vi "test_TrajectoryMH100122AODRAPS.vi"() -> ()   [LabVIEW 2010, in "TrajectoryMH100122AODRAPS.lvclass"]
uses:
  TrajectoryMH100122AODRAPS.lvclass
  raps_points_cluster.ctl
  common/classes/ErrorController/ErrorController/ErrorController.lvclass
  TrajectoryMH100122AODRAPS.lvclass/TrajectoryMH100122AODRAPS.ctl
  common/classes/ErrorController/ErrorController/class_data.vi
panel:
  in  "RAPS points cluster":T1
  out "error loaded?":bool
  in  "Define":bool
  in  "initialise":bool
  in  "number of frames":i32
  in  "startButton":bool
  in  "createButton":bool
  in  "repetition rate":dbl[unit]=10.0
  in  "stop":bool
  # "Test VI for TrajectoryMH100122AODRAPS"
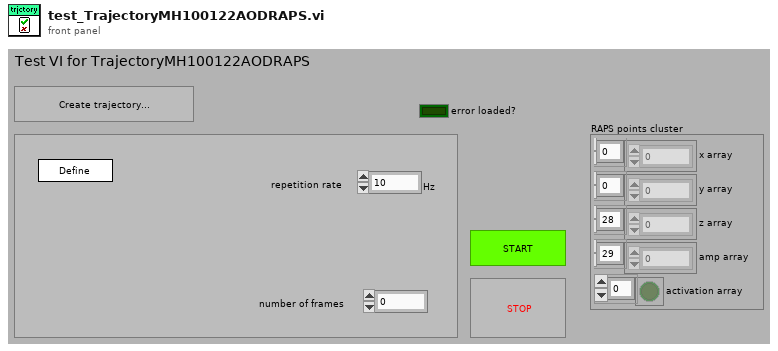
[diagram p1: front panel]
types:
  T1 = typedef "TrajectoryMH100122AODRAPS.lvclass/raps_points_cluster.ctl" = cluster{"x array":u16[], "y array":u16[], "z array":u16[], "amp array":u16[], "activation array":bool[]}
  T2 = typedef "plugin_specification.ctl" = cluster{"class path":string, "configuration":string, "label":string, "settings name":string}
  T3 = typedef "XComponentSpecification.xctl/data.ctl" = cluster{"class path":string, "configuration":string, "label":string, "settings name":string}
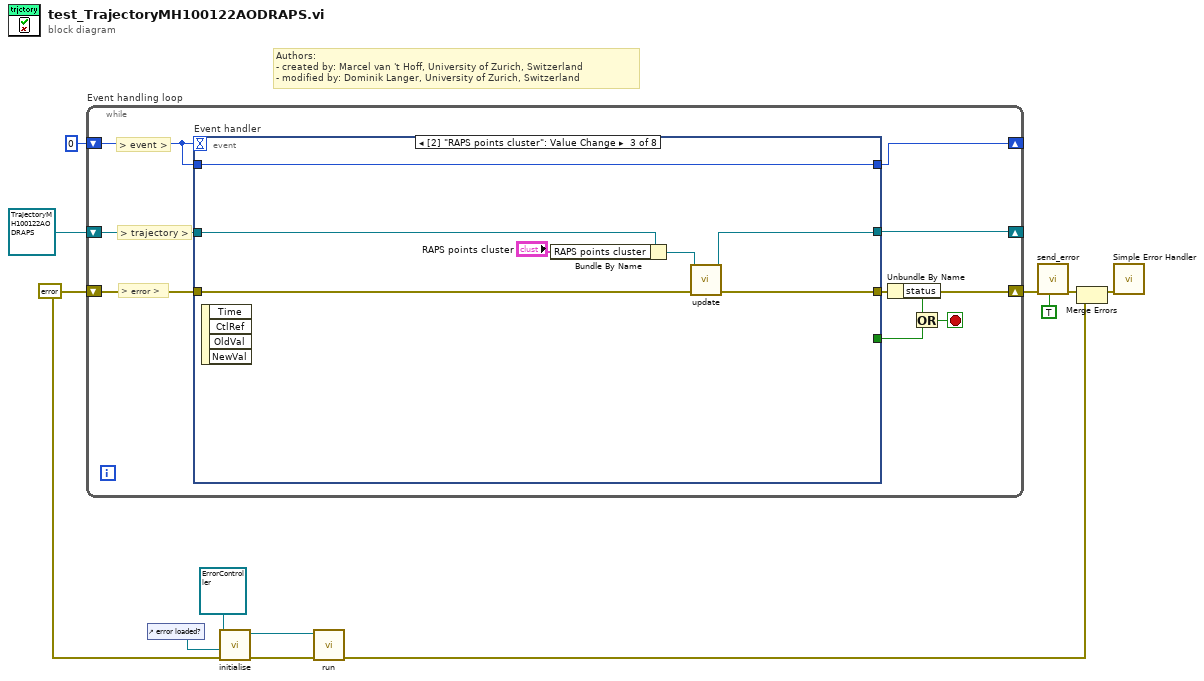
[diagram p0: block diagram]
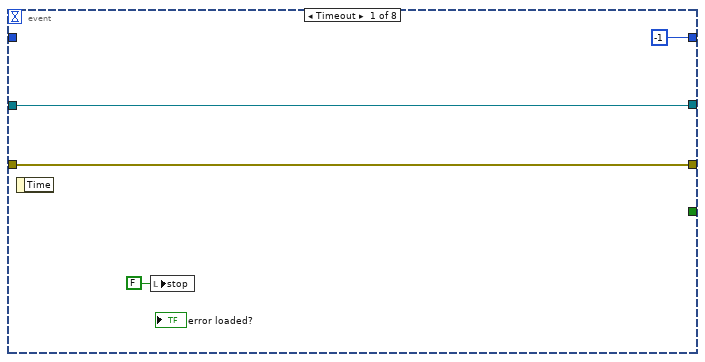
[diagram p2: hidden frame]
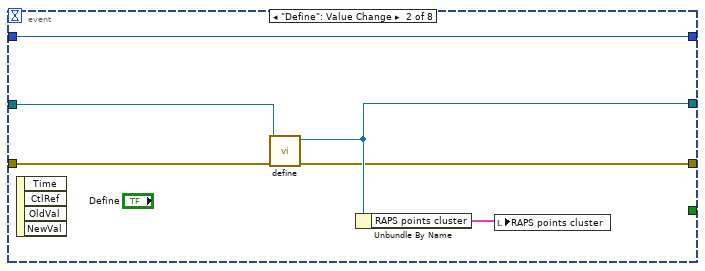
[diagram p3: hidden frame]
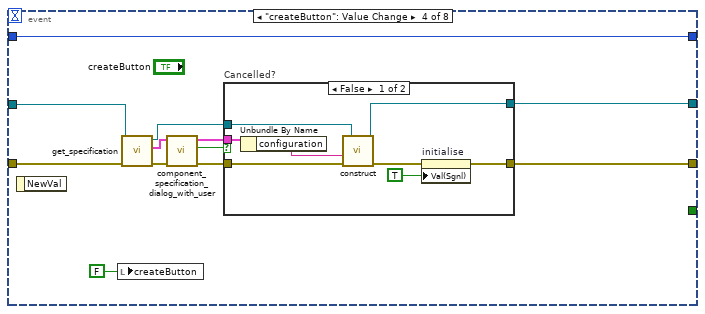
[diagram p4: hidden frame]
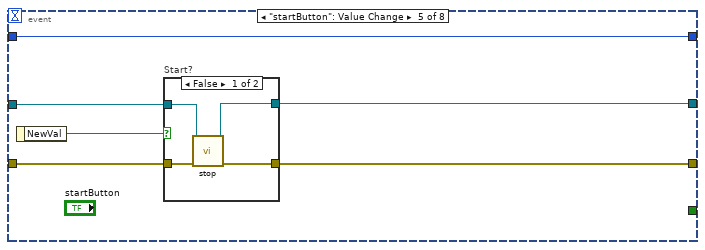
[diagram p6: hidden frame]
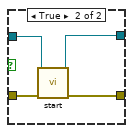
[diagram p7: hidden frame]
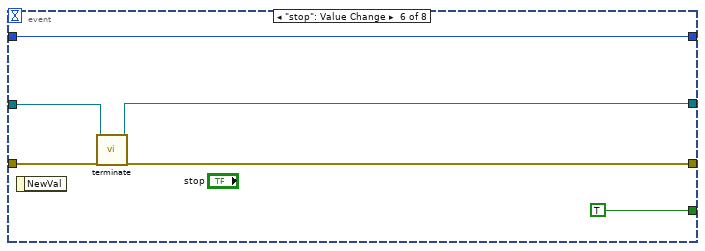
[diagram p8: hidden frame]
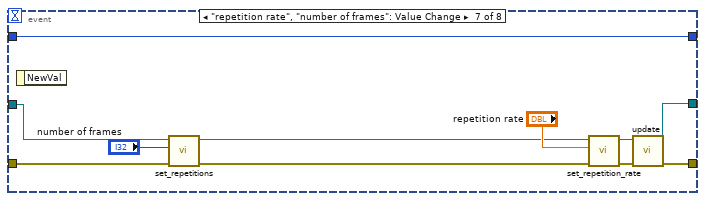
[diagram p9: hidden frame]
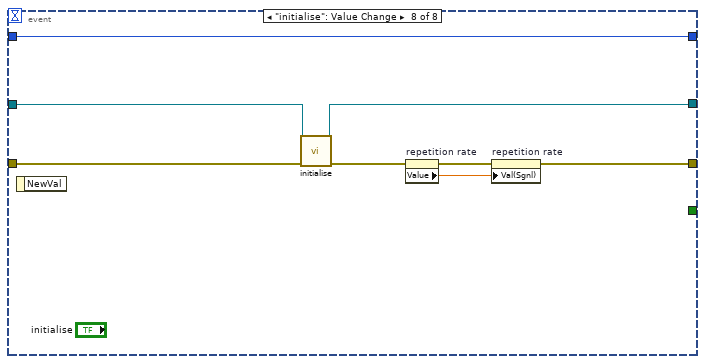
[diagram p10: hidden frame]
diagram:
  w8 = errorcluster {"status"=FALSE, "code"=0, "source"=""} ("error out")
  # "Authors: \n- created by: Marcel van 't Hoff, University of Zurich, Switzerland\n- modified by: Dominik Langer, University of Zurich, Switzerland"
  n1 = while "Event handling loop" {
    shift-right: [w14] -> _
    shift-left: 0 -> [w13]
    shift-right: [w18] -> w3
    shift-left: w8 -> [w21]
    shift-right: [w19] -> _
    shift-left: refnum<class "TrajectoryMH100122AODRAPS.lvclass"> refnum ("TrajectoryMG100122AODFrameScan.lvclass") -> [w20]
    stop <- w16 stop-if-true
    # "> trajectory >"
    # "> error >"
    # "> event >"
    n2 = event "Event handler" shown="[2] \"RAPS points cluster\": Value Change" {
      selector: _ -> [_ _ _ _ _ _ _ _]
      dyn-events: _ -> [_ _ _ _ _ _ _ _]
      timeout: w13 -> [_ _ _ _ _ _ _ _]
      tunnel: [-1 w31 w38 w50 w66 w79 w91 w99] -> w14
      tunnel: w13 -> [_ w31 w38 w50 w66 w79 w91 w99]
      tunnel: [w23 w26 w36 w47 w63 w77 w87 w92] -> w18
      tunnel: w21 -> [w23 w29 w37 w44 w64 w78 w89 w98]
      tunnel: [w24 w27 w35 w48 w62 w75 w86 w96] -> w19
      tunnel: w20 -> [w24 w30 w34 w42 w65 w76 w88 w97]
      tunnel: [_ _ _ _ _ TRUE ("stop") _ _] -> w15
      event Timeout {
        n3 = event-data() -> ()  [unwired: 1 in, 1 out]
        n4 = local write "stop"(FALSE ("stop")) -> ()
      }
      event "Define": Value Change {
        n5 = event-data() -> ()  [unwired: 1 in, 4 out]
        n6 = call-dynamic "define.vi"("error in (no error)"=w29, "TrajectoryMH100122AODRAPS in"=w30) -> ("error out"=w26:errorcluster, "TrajectoryMH100122AODRAPS out"=w27:refnum<class "TrajectoryMH100122AODRAPS.lvclass">)  [unwired: 8 in]
        n7 = Unbundle By Name(w27) -> ("RAPS points cluster"=w28:T1)
        n8 = local write "RAPS points cluster"(w28) -> ()
      }
      event Value Change {
        n9 = event-data() -> ()  [unwired: 1 in, 4 out]
        n10 = Bundle By Name(cluster=w34, "RAPS points cluster"="RAPS points cluster") -> (w33:refnum<class "TrajectoryMH100122AODRAPS.lvclass">)
        n11 = call-dynamic "update.vi"("error in (no error)"=w37, "TrajectoryMG100122AODFrameScan in"=w33) -> ("error out"=w36:errorcluster, "TrajectoryMG100122AODFrameScan out"=w35:refnum<class "TrajectoryMH100122AODRAPS.lvclass">)  [unwired: 8 in]
      }
      event "createButton": Value Change {
        n12 = event-data() -> ()  [unwired: 1 in, 1 out]
        n13 = local write "createButton"(FALSE ("createButton")) -> ()
        n14 = call-dynamic "get_specification.vi"("error in (no error)"=w44, "GenericPlugin in"=w42) -> ("error out"=w45:errorcluster, "component specification"=w46:T2, "GenericPlugin out"=w41:refnum<class "TrajectoryMH100122AODRAPS.lvclass">)  [unwired: 6 in, 1 out]
        n15 = call "component_specification_dialog_with_user.vi"("error in (no error)"=w45, "component specification in"=w46) -> ("error out"=w43:errorcluster, "cancelled?"=w39:bool, "component specification out"=w40:T3)  [unwired: 7 in]
        n16 = case "Cancelled?" shown="False" w39 {
          tunnel: [w58 w59] -> w48
          tunnel: [w55 w60] -> w47
          tunnel: w43 -> [w54 w60]
          tunnel: w41 -> [w53 w59]
          tunnel: w40 -> [w52 _]
          frame False {
            n17 = Unbundle By Name(w52) -> ("configuration"=w51:string)
            n18 = call-dynamic "construct.vi"("error in (no error)"=w54, "configuration name"=w51, "GenericPlugin in"=w53) -> ("error out"=w56:errorcluster, "GenericPlugin out"=w58:refnum<class "TrajectoryMH100122AODRAPS.lvclass">)  [unwired: 7 in]
            n19 = property on="initialise" class="Bool (strict)"(error in=w56, "Val(Sgnl)"=TRUE ("Value (Signaling)")) -> (error out=w55:errorcluster)  [unwired: 1 in, 1 out]
          }
          frame True {
          }
        }
      }
      event "startButton": Value Change {
        n20 = event-data() -> ("NewVal"=w61:bool)  [unwired: 1 in]
        n21 = case "Start?" shown="False" w61 {
          tunnel: w65 -> [w68 w74]
          tunnel: w64 -> [w70 w73]
          tunnel: [w69 w72] -> w63
          tunnel: [w67 w71] -> w62
          frame False {
            n22 = call-dynamic "stop.vi"("error in (no error)"=w70, "TrajectoryMG100122GenericFPGA in"=w68) -> ("error out"=w69:errorcluster, "TrajectoryMG100122GenericFPGA out"=w67:refnum<class "TrajectoryMH100122AODRAPS.lvclass">)  [unwired: 8 in]
          }
          frame True {
            n23 = call-dynamic "start.vi"("error in (no error)"=w73, "TrajectoryMG100122GenericFPGA in"=w74) -> ("error out"=w72:errorcluster, "TrajectoryMG100122GenericFPGA out"=w71:refnum<class "TrajectoryMH100122AODRAPS.lvclass">)  [unwired: 8 in]
          }
        }
      }
      event "stop": Value Change {
        n24 = event-data() -> ()  [unwired: 1 in, 1 out]
        n25 = call-dynamic "terminate.vi"("error in (no error)"=w78, "GenericPlugin in"=w76) -> ("error out"=w77:errorcluster, "GenericPlugin out"=w75:refnum<class "TrajectoryMH100122AODRAPS.lvclass">)  [unwired: 8 in]
      }
      event "repetition rate", "number of frames": Value Change {
        n26 = event-data() -> ()  [unwired: 1 in, 1 out]
        n27 = call-dynamic "set_repetitions.vi"("error in (no error)"=w89, "repetitions"="number of frames", "GenericTrajectory in"=w88) -> ("error out"=w85:errorcluster, "GenericTrajectory out"=w83:refnum<class "TrajectoryMH100122AODRAPS.lvclass">)  [unwired: 7 in]
        n28 = call-dynamic "set_repetition_rate.vi"("error in (no error)"=w85, "repetition rate"="repetition rate", "TrajectoryMH100122AODRAPS in"=w83) -> ("error out"=w81:errorcluster, "TrajectoryMH100122AODRAPS out"=w82:refnum<class "TrajectoryMH100122AODRAPS.lvclass">)  [unwired: 7 in]
        n29 = call-dynamic "update.vi"("error in (no error)"=w81, "TrajectoryMG100122AODFrameScan in"=w82) -> ("error out"=w87:errorcluster, "TrajectoryMG100122AODFrameScan out"=w86:refnum<class "TrajectoryMH100122AODRAPS.lvclass">)  [unwired: 8 in]
      }
      event "initialise": Value Change {
        n30 = event-data() -> ()  [unwired: 1 in, 1 out]
        n31 = call-dynamic "initialise.vi"("error in (no error)"=w98, "GenericPlugin in"=w97) -> ("error out"=w93:errorcluster, "GenericPlugin out"=w96:refnum<class "TrajectoryMH100122AODRAPS.lvclass">)  [unwired: 8 in]
        n32 = property on="repetition rate" class="DigNum (strict)"(error in=w93) -> (error out=w94:errorcluster, "Value"=w95:dbl[unit])  [unwired: 1 in, 1 out]
        n33 = property on="repetition rate" class="DigNum (strict)"(error in=w94, "Val(Sgnl)"=w95) -> (error out=w92:errorcluster)  [unwired: 1 in, 1 out]
      }
    }
    n34 = Unbundle By Name(w18) -> ("status"=w17:bool)
    n35 = Or(x=w17, y=w15) -> (x .or. y?=w16:bool)
  }
  n36 = control-ref of="error loaded?"() -> (w9:refnum<vi>)
  n37 = call-dynamic "initialise.vi"("error in (no error)"=w8, "error boolean"=w9, "ErrorController in"=refnum<class "ErrorController.lvclass"> refnum ("ErrorController.lvclass")) -> ("error out"=w6:errorcluster, "ErrorController out"=w7:refnum<class "ErrorController.lvclass">)  [unwired: 7 in]
  n38 = call "run.vi"("error in (no error)"=w6, "ErrorController in"=w7) -> ("error out"=w2:errorcluster)  [unwired: 8 in, 1 out]
  n39 = call "send_error.vi"("last error? (F)"=TRUE, "error in (no error)"=w3) -> ("error out"=w4:errorcluster)  [unwired: 9 in]
  n40 = Merge Errors(w4, w2) -> (w1:errorcluster)
  n41 = call <vilib>:"Simple Error Handler.vi"("error in (no error)"=w1) -> ()  [unwired: 4 in, 5 out]
